vi "set initial state.vi"(10 "state module configuration.initial state":u8, 11 "tag bus configurable plugin module configuration in":refnum<class "TEST CONFIGURATION.lvclass">) -> (3 "tag bus configurable plugin module configuration out":refnum<class "TEST CONFIGURATION.lvclass">)   [LabVIEW 2013, in "configuration tests.lvlib" / "TEST CONFIGURATION.lvclass"]
uses:
  TEST CONFIGURATION.lvclass
  TEST CONFIGURATION.lvclass/TEST CONFIGURATION.ctl
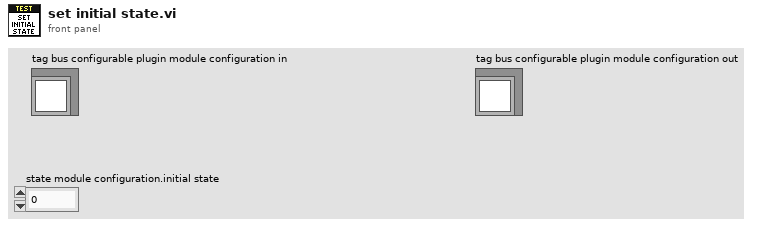
[diagram p1: front panel]
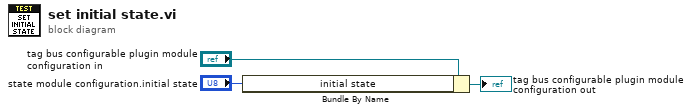
[diagram p0: block diagram]
diagram:
  n1 = Bundle By Name(cluster="tag bus configurable plugin module configuration in", "initial state"="state module configuration.initial state") -> (→"tag bus configurable plugin module configuration out":refnum<class "TEST CONFIGURATION.lvclass">)
